vi "Digitizer1_FGV.vi"(8 "error in (no error)":errorcluster, 9 "Operation (Read)":enum16{"Write", "Read"}(ring)=enum."Read", 11 "Write data":refnum<k15>="PXI1Slot3" caption="handles in") -> (0 "error out":errorcluster, 3 "Read data":refnum<k15>)   [LabVIEW 2020]
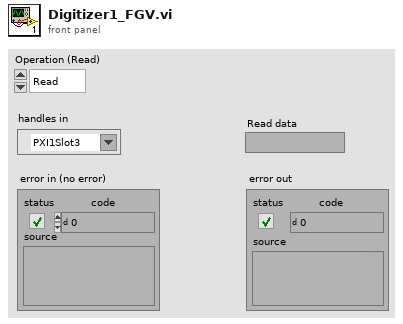
[diagram p1: front panel]
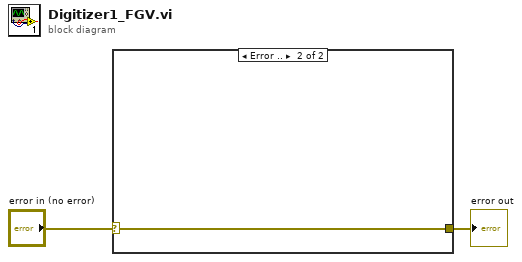
[diagram p0: block diagram]
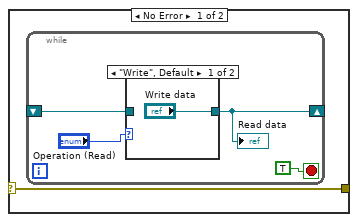
[diagram p2: hidden frame]
diagram:
  n1 = case shown="Error .." "error in (no error)" {
    selector: "error in (no error)" -> [w3 w10]
    tunnel: [w3 w10] -> w1
    frame No Error {
      n2 = while {
        shift-right: [w5] -> _
        shift-left: _ -> [w4]
        stop <- TRUE stop-if-true
        n3 = case shown="\"Write\", Default" "Operation (Read)" {
          tunnel: ["Write data" w9] -> w5
          tunnel: w4 -> [_ w9]
          frame "Write", Default {
          }
          frame "Read" {
          }
        }
        "Read data" <- w5
      }
    }
    frame Error {
    }
  }
  "error out" <- w1
